vi "Publish Instrument Error.vi"(8 "error in (no error)":errorcluster, 9 "Instrument String":string, 10 "Instrument Msg":refnum<class "Instrument Msg.lvclass">, 11 "Actor in":refnum<class "Actor.lvclass">) -> (0 "error out":errorcluster, 3 "Actor out":refnum<class "Actor.lvclass">)   [LabVIEW 2020, in "Instrument Handler.lvlib"]
doc: "Publish Instrument error data."
uses:
  Instrument Handler.lvlib
  PPL/HDH.Actor Framework.Core.Actor.lvlibp/1abvi3w/vi.lib/ActorFramework/Actor/Actor.lvclass
  Messages/Instrument Msg/Instrument Msg.lvclass
  PPL/HDH.Actor Framework.Core.Actor.lvlibp/1abvi3w/vi.lib/ActorFramework/Message Enqueuer/Message Priority.ctl
  Data/Instrument Error Data/Instrument Error Data.lvclass/Instrument Error Data.ctl
  Data/Instrument Error Data/Instrument Error Data.lvclass
  PPL/HDH.Actor Framework.Core.Publisher.lvlibp/Publisher Messages/Publish Msg/Publish Msg.lvclass
  PPL/HDH.Data.Generic.lvlibp
  PPL/HDH.Actor Framework.Core.Actor.lvlibp/1abvi3w/vi.lib/ActorFramework/Message Enqueuer/Message Enqueuer.lvclass
  C:/Current projects/WS/PPL/HDH.Data.Generic.lvlibp/Data.lvclass
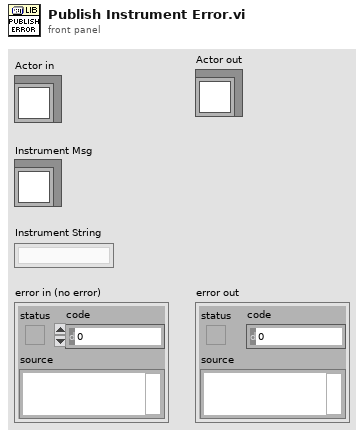
[diagram p1: front panel]
types:
  T1 = typedef "HDH.Actor Framework.Core.Actor.lvlibp/Message Enqueuer.lvclass/Message Priority.ctl" = enum16{"Low", "Normal", "High"}
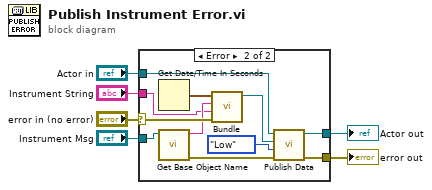
[diagram p0: block diagram]
diagram:
  n1 = case shown="Error" "error in (no error)" {
    selector: "error in (no error)" -> [w7 w16]
    tunnel: [w8 w18] -> w5
    tunnel: "Actor in" -> [w8 w19]
    tunnel: "Instrument Msg" -> [_ w15]
    tunnel: "Instrument String" -> [_ w13]
    tunnel: [w7 w9] -> w1
    frame No Error {
    }
    frame Error {
      n2 = Get Date/Time In Seconds() -> (seconds since 1Jan1904=w17:timestamp)
      n3 = call "Get Base Object Name.vi"("Object in"=w15) -> ("error out"=w10:errorcluster, "Base class name"=w14:string)  [unwired: 9 in]
      n4 = call "Bundle.vi"("error in"=w16, "Instrument String"=w13, "Msg Name"=w14, "Time Stamp"=w17) -> ("Instrument Error Data out"=w11:refnum<class "Instrument Error Data.lvclass">)  [unwired: 7 in]
      n5 = call "Publish Data.vi"("error in (no error)"=w10, "Message Priority (Normal)"=Message_Priority."Low", "Data to Publish"=w11, "Actor in"=w19) -> ("error out"=w9:errorcluster, "Actor out"=w18:refnum<class "Actor.lvclass">)  [unwired: 5 in, 1 out]
    }
  }
  "Actor out" <- w5
  "error out" <- w1
